vi "cuartocalculadora.vi"() -> ()   [LabVIEW 2012]
panel:
  out "Multiplica":dbl
  out "Divide":dbl
  out "Resta":dbl
  out "Suma":dbl
  in  "B":dbl
  in  "A":dbl
  in  "stop":bool
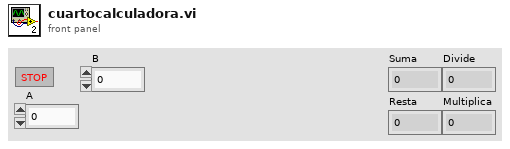
[diagram p1: front panel]
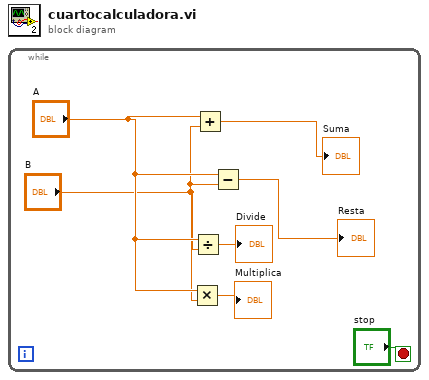
[diagram p0: block diagram]
diagram:
  n1 = while {
    stop <- "stop" stop-if-true
    n2 = Multiply(x="A", y="B") -> (x*y=→"Multiplica":dbl)
    n3 = Divide(x="A", y="B") -> (x/y=→"Divide":dbl)
    n4 = Add(x="A", y="B") -> (x+y=→"Suma":dbl)
    n5 = Subtract(x="A", y="B") -> (x-y=→"Resta":dbl)
  }
